vi "Draw_rectangles_near_rounded_corners.vi"(8 "error in (no error)":errorcluster, 9 "Inner box coords":T1, 10 "Outer box coords":T1, 11 "Refnum in":T2) -> (0 "error out":errorcluster, 3 "Refnum out":T2)   [LabVIEW 2018, in "Cage Diagram.lvlib"]
uses:
  Cage Diagram.lvlib
  <vilib>/vision/Image Controls.llb/IMAQ Image.ctl
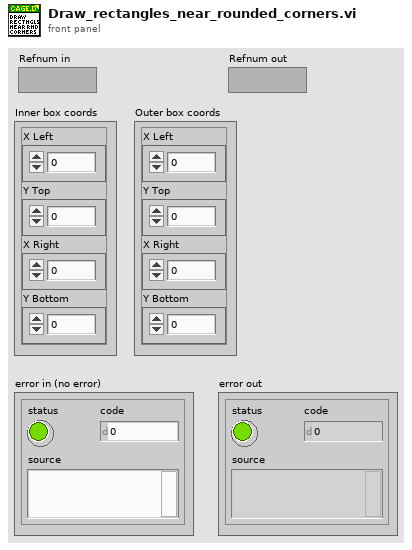
[diagram p1: front panel]
types:
  T1 = cluster{"X Left":dbl, "Y Top":dbl, "X Right":dbl, "Y Bottom":dbl}
  T2 = typedef "IMAQ Image.ctl" = refnum<image>
  T3 = cluster{"X Left":dbl, dbl, "X Right":dbl, "Y Bottom":dbl}
  T4 = cluster{"X Right":dbl, "Y Top":dbl, dbl, "Y Bottom":dbl}
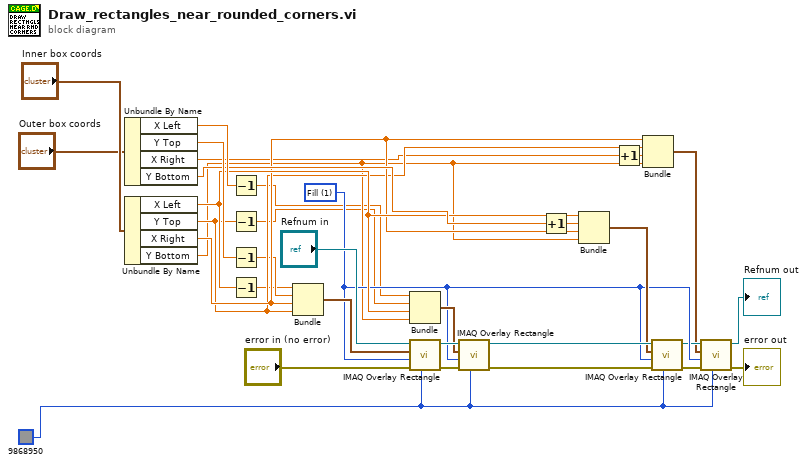
[diagram p0: block diagram]
diagram:
  w1 = u32 9868950 ("Color")
  w17 = u32 1 items=["Frame", "Fill", "Highlight"] ("Drawing Mode (Frame)")
  n1 = Unbundle By Name("Outer box coords") -> ("X Left"=w20:dbl, "Y Top"=w27:dbl, "X Right"=w9:dbl, "Y Bottom"=w19:dbl)
  n2 = Unbundle By Name("Inner box coords") -> ("X Left"=w18:dbl, "Y Top"=w10:dbl, "X Right"=w11:dbl, "Y Bottom"=w8:dbl)
  n3 = Decrement(x=w20) -> (x-1=w5:dbl)
  n4 = Decrement(x=w10) -> (x-1=w4:dbl)
  n5 = Decrement(x=w27) -> (x-1=w7:dbl)
  n6 = Decrement(x=w18) -> (x-1=w6:dbl)
  n7 = Bundle(w6, w7, "X Right"=w11, "Y Top"=w10) -> (w28:cluster{dbl, dbl, "X Right":dbl, "Y Top":dbl})  [unwired: 1 in]
  n8 = Bundle(w5, w4, "X Left"=w18, "Y Bottom"=w8) -> (w24:cluster{dbl, dbl, "X Left":dbl, "Y Bottom":dbl})  [unwired: 1 in]
  n9 = call "IMAQ Overlay Rectangle"("Color"=w1, "error in (no error)"="error in (no error)", "Drawing Mode (Frame)"=w17, "Rectangle"=w28, "Image"="Refnum in") -> ("error out"=w26:errorcluster, "Image Out"=w25:T2)  [unwired: 5 in]
  n10 = call "IMAQ Overlay Rectangle"("Color"=w1, "error in (no error)"=w26, "Drawing Mode (Frame)"=w17, "Rectangle"=w24, "Image"=w25) -> ("error out"=w23:errorcluster, "Image Out"=w22:T2)  [unwired: 5 in]
  n11 = Increment(x=w19) -> (x+1=w3:dbl)
  n12 = Bundle("X Left"=w18, w3, "X Right"=w11, "Y Bottom"=w8) -> (w21:T3)  [unwired: 1 in]
  n13 = Increment(x=w9) -> (x+1=w2:dbl)
  n14 = Bundle("X Right"=w11, "Y Top"=w10, w2, "Y Bottom"=w8) -> (w12:T4)  [unwired: 1 in]
  n15 = call "IMAQ Overlay Rectangle"("Color"=w1, "error in (no error)"=w23, "Drawing Mode (Frame)"=w17, "Rectangle"=w21, "Image"=w22) -> ("error out"=w16:errorcluster, "Image Out"=w15:T2)  [unwired: 5 in]
  n16 = call "IMAQ Overlay Rectangle"("Color"=w1, "error in (no error)"=w16, "Drawing Mode (Frame)"=w17, "Rectangle"=w12, "Image"=w15) -> ("error out"=→"error out":errorcluster, "Image Out"=→"Refnum out":T2)  [unwired: 5 in]
